vi "ISO Week Number.vi"() -> (0 "seconds (now)":dbl format="%<%X\n%x>T", 1 "ISO date":T1, 2 "ISO week":i32)   [LabVIEW 2014]
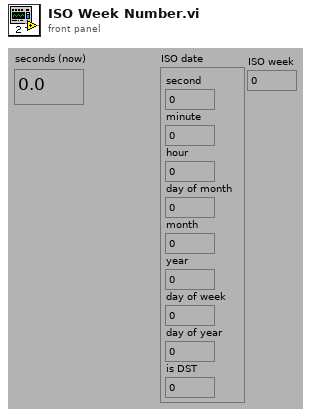
[diagram p1: front panel]
types:
  T1 = cluster{"second":i32, "minute":i32, "hour":i32, "day of month":i32, "month":i32, "year":i32, "day of week":i32, "day of year":i32, "is DST":i32}
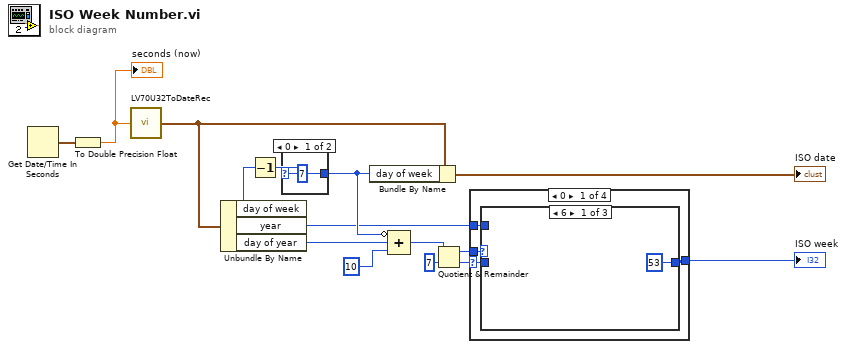
[diagram p0: block diagram]
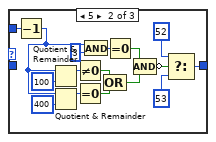
[diagram p2: hidden frame]
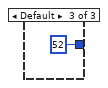
[diagram p3: hidden frame]
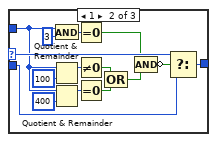
[diagram p6: hidden frame]
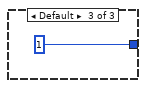
[diagram p7: hidden frame]
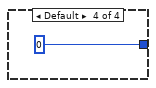
[diagram p8: hidden frame]
diagram:
  n1 = Get Date/Time In Seconds() -> (seconds since 1Jan1904=w2:timestamp)
  n2 = To Double Precision Float(number=w2) -> (double precision float=w1:dbl)
  "seconds (now)" <- w1
  n3 = call <vilib>:"LV70U32ToDateRec.vi"("Time"=w1) -> ("date time rec"=w15:T1)
  n4 = Unbundle By Name(w15) -> ("day of week"=w9:i32, "year"=w4:i32, "day of year"=w3:i32)
  n5 = Decrement(x=w9) -> (x-1=w10:i32)
  n6 = case shown="0" w10 {
    selector: w10 -> [_ w17]
    tunnel: [7 ("day of week") w17] -> w8
    frame 0 {
    }
    frame Default {
    }
  }
  n7 = Bundle By Name(cluster=w15, "day of week"=w8) -> (→"ISO date":T1)
  n8 = Compound Arithmetic op=ADD(invert w8, w3, 10 ("Input")) -> (w12:i32)
  n9 = Quotient & Remainder(x=w12, y=7) -> (x-y*floor(x/y)=w6:i32, floor(x/y)=w7:i32)
  n10 = case shown="0" w7 {
    selector: w7 -> [w21 w40 w42 _]
    tunnel: [w19 w40 w43 0] -> w5
    tunnel: w6 -> [w20 _ w44 _]
    tunnel: w4 -> [w18 _ w41 _]
    frame 0 {
      n11 = case shown="6" w20 {
        tunnel: [53 w38 52 ("t")] -> w19
        tunnel: w21 -> [_ _ _]
        tunnel: w18 -> [_ w23 _]
        frame 6 {
        }
        frame 5 {
          n12 = Decrement(x=w23) -> (x-1=w26:i32)
          n13 = Quotient & Remainder(x=w26, y=100) -> (x-y*floor(x/y)=w35:i32)  [unwired: 1 out]
          n14 = Quotient & Remainder(x=w26, y=400) -> (x-y*floor(x/y)=w36:i32)  [unwired: 1 out]
          n15 = Not Equal To 0?(x=w35) -> (x != 0?=w30:bool)
          n16 = Equal To 0?(x=w36) -> (x = 0?=w29:bool)
          n17 = And(x=w26, y=3) -> (x .and. y?=w34:i32)
          n18 = Compound Arithmetic op=OR(w30, w29) -> (w28:bool)
          n19 = Equal To 0?(x=w34) -> (x = 0?=w37:bool)
          n20 = Compound Arithmetic op=AND(w37, w28) -> (invert w31:bool)
          n21 = Select(t=52, s=w31, f=53 ("t")) -> (s? t:f=w38:i32)
        }
        frame Default {
        }
      }
    }
    frame 1..52 {
    }
    frame 53 {
      n22 = case shown="0" w44 {
        selector: w44 -> [_ w59 _]
        tunnel: [w45 w60 1] -> w43
        tunnel: w42 -> [w45 w58 _]
        tunnel: w41 -> [_ w46 _]
        frame 0 {
        }
        frame 1 {
          n23 = And(x=w46, y=3) -> (x .and. y?=w54:i32)
          n24 = Quotient & Remainder(x=w46, y=100) -> (x-y*floor(x/y)=w55:i32)  [unwired: 1 out]
          n25 = Quotient & Remainder(x=w46, y=400) -> (x-y*floor(x/y)=w56:i32)  [unwired: 1 out]
          n26 = Equal To 0?(x=w54) -> (x = 0?=w57:bool)
          n27 = Not Equal To 0?(x=w55) -> (x != 0?=w49:bool)
          n28 = Equal To 0?(x=w56) -> (x = 0?=w48:bool)
          n29 = Compound Arithmetic op=OR(w49, w48) -> (w47:bool)
          n30 = Compound Arithmetic op=AND(w57, w47) -> (invert w50:bool)
          n31 = Select(t=w59, s=w50, f=w58) -> (s? t:f=w60:i32)
        }
        frame Default {
        }
      }
    }
    frame Default {
    }
  }
  "ISO week" <- w5
